vi "send refresh.vi"(11 "User Event in":T1) -> ()   [LabVIEW 2013, in "PL Framework Configuration Tool.lvlib" / "Engine Mappings.lvclass"]
uses:
  Engine Mappings.lvclass
  <vilib>/NI/CEF/CEF_TreeControl/Node/UserEventRef.ctl
  <vilib>/NI/CEF/CEF_TreeControl/Controls/EventCluster.ctl
  <vilib>/NI/CEF/CEF_TreeControl/NISE_CEF_TreeControl.lvlib
  <vilib>/NI/CEF/CEF_TreeControl/Node/NISE_CEF_Node.lvclass
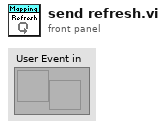
[diagram p1: front panel]
types:
  T1 = typedef "NISE_CEF_Node.lvclass/UserEventRef.ctl" = refnum<user-event>
  T2 = typedef "NISE_CEF_TreeControl.lvlib/EventCluster.ctl" = cluster{"command":string, "data":string}
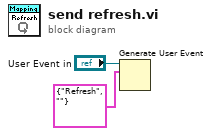
[diagram p0: block diagram]
diagram:
  n1 = Generate User Event(user event="User Event in", event data cluster=T2 {"command"="Refresh", "data"=""} ("event data")) -> ()  [unwired: 2 in, 2 out]
